vi "AutonSelector.vi"(10 "Buttons1":T1, 11 "Buttons in":T1) -> ()   [LabVIEW 2013]
uses:
  <vilib>/Rock Robotics/WPI/Joystick/WPI_JoystickButtonState.ctl
  Robot Global Data.vi
panel:
  out "Current File":string
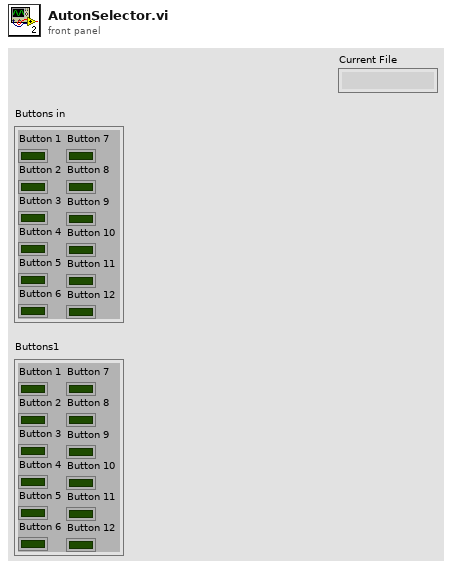
[diagram p1: front panel]
types:
  T1 = typedef "WPI_JoystickButtonState.ctl" = cluster{"Button 1":bool, "Button 2":bool, "Button 3":bool, "Button 4":bool, "Button 5":bool, "Button 6":bool, "Button 7":bool, "Button 8":bool, "Button 9":bool, "Button 10":bool, "Button 11":bool, "Button 12":bool}
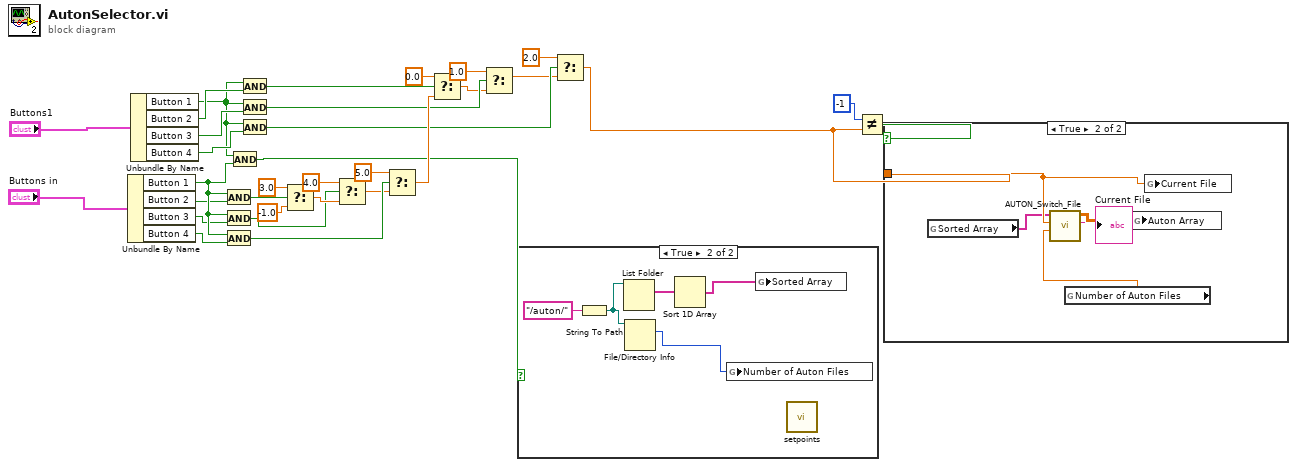
[diagram p0: block diagram]
diagram:
  n1 = Unbundle By Name("Buttons in") -> ("Button 1"=w4:bool, "Button 2"=w2:bool, "Button 3"=w3:bool, "Button 4"=w5:bool)
  n2 = Unbundle By Name("Buttons1") -> ("Button 1"=w23:bool, "Button 2"=w24:bool, "Button 3"=w25:bool, "Button 4"=w26:bool)
  n3 = And(x=w4, y=w2) -> (x .and. y?=w6:bool)
  n4 = And(x=w4, y=w3) -> (x .and. y?=w9:bool)
  n5 = And(x=w4, y=w5) -> (x .and. y?=w15:bool)
  n6 = And(x=w23, y=w4) -> (x .and. y?=w13:bool)
  n7 = And(x=w23, y=w24) -> (x .and. y?=w22:bool)
  n8 = And(x=w23, y=w25) -> (x .and. y?=w20:bool)
  n9 = And(x=w23, y=w26) -> (x .and. y?=w27:bool)
  n10 = Select(t=3.0, s=w6, f=-1.0) -> (s? t:f=w10:dbl)
  n11 = Select(t=4.0, s=w9, f=w10) -> (s? t:f=w12:dbl)
  n12 = Select(t=5.0, s=w15, f=w12) -> (s? t:f=w28:dbl)
  n13 = Select(t=0.0, s=w22, f=w28) -> (s? t:f=w19:dbl)
  n14 = Select(t=1.0, s=w20, f=w19) -> (s? t:f=w17:dbl)
  n15 = case shown="True" w13 {
    frame False {
    }
    frame True {
      n16 = String To Path(string="/auton/") -> (path=w36:path)
      n17 = List Folder(path=w36) -> (filenames=w35:string[])  [unwired: 3 in, 3 out]
      n18 = File/Directory Info(path=w36) -> (size=w33:i64)  [unwired: 1 in, 6 out]
      n19 = Sort 1D Array(array=w35) -> (sorted array=w34:string[])
      n20 = global write "Robot Global Data.vi" "Number of Auton Files"(w33) -> ()
      n21 = global write "Robot Global Data.vi" "Sorted Array"(w34) -> ()
      n22 = call "setpoints.vi"() -> ()  [unwired: 12 in]
    }
  }
  n23 = Select(t=2.0, s=w27, f=w17) -> (s? t:f=w29:dbl)
  n24 = Not Equal?(x=-1, y=w29) -> (x != y?=w30:bool)
  n25 = case shown="True" w30 {
    tunnel: w29 -> [_ w41]
    frame False {
    }
    frame True {
      n26 = global read "Robot Global Data.vi" "Sorted Array"() -> (w38:string[])
      n27 = global read "Robot Global Data.vi" "Number of Auton Files"() -> (w39:dbl)
      n28 = call "AUTON_Switch_File.vi"("Number of Auton Files"=w39, "Auton File"=w41, "Auton Files"=w38) -> ("Current File"=→"Current File":string, "Auton Array"=w42:dbl[][])  [unwired: 7 in]
      n29 = global write "Robot Global Data.vi" "Auton Array"(w42) -> ()
      n30 = global write "Robot Global Data.vi" "Current File"(w41) -> ()
    }
  }
